vi "Filename Generate.vi"(0 "TR Number":string, 5 "Serial Number":string) -> (4 "Hist File Path":path, 6 "Filename for Hist data":string, 8 "Sample file Path":path, 10 "Filename for Samples":string)   [LabVIEW 2009]
uses:
  Globals Wilt.vi
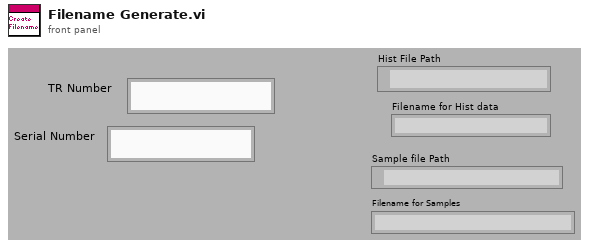
[diagram p1: front panel]
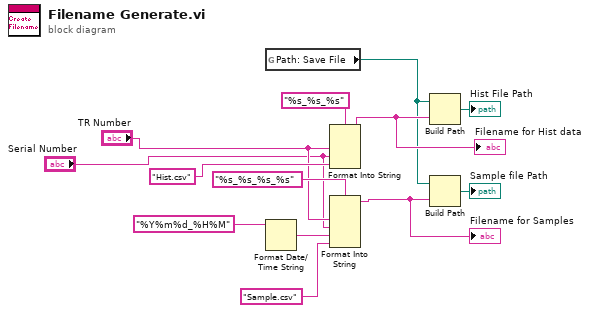
[diagram p0: block diagram]
diagram:
  n1 = global read "Globals Wilt.vi" "Path: Save File"() -> (w12:path)
  n2 = Format Date/Time String(time format string (%c)="%Y%m%d_%H%M") -> (date/time string=w11:string)  [unwired: 2 out]
  n3 = Format Into String(format string="%s_%s_%s", "TR Number", "Serial Number", "Hist.csv" ("input 2")) -> (resulting string=w13:string)  [unwired: 2 in, 1 out]
  "Filename for Hist data" <- w13
  n4 = Format Into String(format string="%s_%s_%s_%s", "TR Number", "Serial Number", w11, "Sample.csv" ("input 4")) -> (resulting string=w3:string)  [unwired: 2 in, 1 out]
  "Filename for Samples" <- w3
  n5 = Build Path(base path=w12, name or relative path=w13) -> (appended path=→"Hist File Path":path)
  n6 = Build Path(base path=w12, name or relative path=w3) -> (appended path=→"Sample file Path":path)
